vi "make_temp_files.vi"() -> ()   [LabVIEW 2012]
panel:
  in  "error in":errorcluster
  out "error out":errorcluster
  in  "Destination Path":path
  out "Number of Files found":i32
  in  "Source Path":path
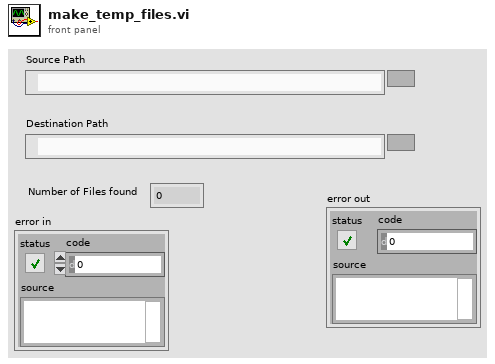
[diagram p1: front panel]
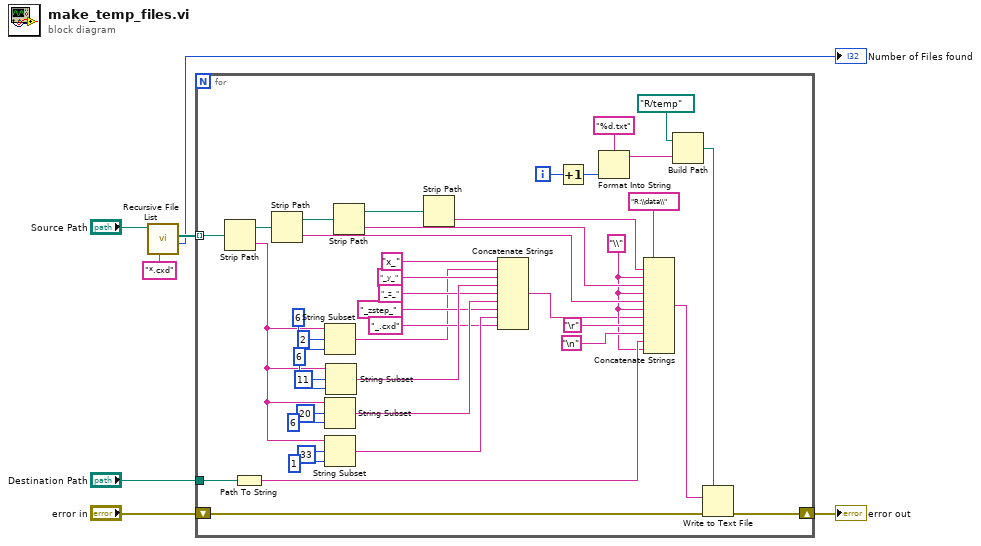
[diagram p0: block diagram]
diagram:
  n1 = call <vilib>:"Recursive File List.vi"("pattern"="*.cxd", "Folder Path"="Source Path") -> ("Number of Files"=→"Number of Files found":i32, "All Files in Dir"=w6:path[])  [unwired: 5 in, 3 out]
  n2 = for {
    tunnel: w6 -> [w22] mode=indexing
    tunnel: "Destination Path" -> [w16]
    shift-right: [w8] -> w1
    shift-left: "error in" -> [w9]
    i -> [w19]
    w13 = "\\" ("string")
    n3 = Strip Path(path=w22) -> (stripped path=w31:path, name=w36:string)
    n4 = Path To String(path=w16) -> (string=w15:string)
    n5 = Strip Path(path=w31) -> (stripped path=w30:path, name=w14:string)
    n6 = String Subset(string=w36, offset (0)=2, length (rest)=6 ("length (rest)")) -> (substring=w10:string)
    n7 = String Subset(string=w36, offset (0)=20, length (rest)=6 ("length (rest)")) -> (substring=w38:string)
    n8 = String Subset(string=w36, offset (0)=33, length (rest)=1 ("length (rest)")) -> (substring=w34:string)
    n9 = String Subset(string=w36, offset (0)=11, length (rest)=6 ("length (rest)")) -> (substring=w40:string)
    n10 = Strip Path(path=w30) -> (stripped path=w29:path, name=w27:string)
    n11 = Strip Path(path=w29) -> (name=w28:string)  [unwired: 1 out]
    n12 = Concatenate Strings("x_" ("string"), w10, "_y_" ("string"), w40, "_z_" ("string"), w38, "_zstep_" ("string"), w34, "_.cxd" ("string")) -> (w12:string)
    n13 = Increment(x=w19) -> (x+1=w25:i32)
    n14 = Format Into String(format string="%d.txt", w25) -> (resulting string=w24:string)  [unwired: 2 in, 1 out]
    n15 = Concatenate Strings("R:\\data\\" ("string"), w28, w13, w27, w13, w14, w13, w12, "\r", "\n", w15, w13) -> (w20:string)
    n16 = Build Path(base path=path "R:/temp" ("file path (use dialog)"), name or relative path=w24) -> (appended path=w21:path)
    n17 = Write to Text File(file (use dialog)=w21, text=w20, error in=w9) -> (error out=w8:errorcluster)  [unwired: 1 in, 2 out]
  }
  "error out" <- w1
